vi "Get User Input.vi"(9 "Location":u32(ring) items=["None", "Austin, TX", "New York City, NY", "Chicago, IL"], 10 "Gender":enum32{"Radio Selection 1", "Radio Selection 2"}(radio), 11 "Name":string) -> (1 "Location":u32(ring) items=["Austin, TX", "New York City, NY", "Chicago, IL"], 2 "Gender":enum32{"Radio Selection 1", "Radio Selection 2"}(ring), 3 "Name":string)   [LabVIEW 2021, in "Dialog Box UI.lvlib"]
uses:
  Dialog Box UI.lvlib
panel:
  in  "Cancel":bool
  in  "OK":bool
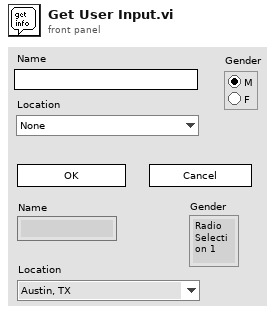
[diagram p1: front panel]
types:
  T1 = enum32{"None", "Radio Selection 1", "Radio Selection 2"}
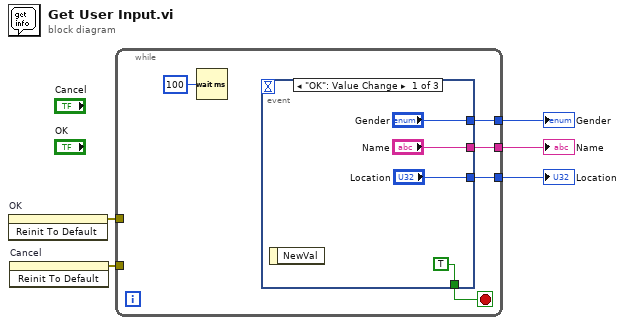
[diagram p0: block diagram]
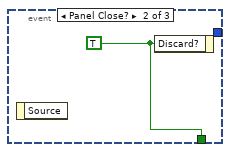
[diagram p2: hidden frame]
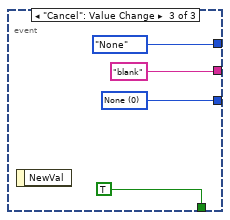
[diagram p3: hidden frame]
diagram:
  n1 = invoke on="OK" class="Bool" method="Reinit To Default"() -> (error out=w4:errorcluster)  [unwired: 3 in, 2 out]
  n2 = invoke on="Cancel" class="Bool" method="Reinit To Default"() -> (error out=w3:errorcluster)  [unwired: 3 in, 2 out]
  n3 = while {
    tunnel: [w10] -> w2
    tunnel: [w9] -> w5
    tunnel: [w8] -> w1
    tunnel: w4 -> [_]
    tunnel: w3 -> [_]
    stop <- w7 stop-if-true
    n4 = Wait (ms)(milliseconds to wait=u32 100) -> ()  [unwired: 1 out]
    n5 = event shown="[0] \"OK\": Value Change" {
      selector: _ -> [_ _ _]
      dyn-events: _ -> [_ _ _]
      timeout: _ -> [_ _ _]
      tunnel: [TRUE w15 TRUE] -> w7
      tunnel: ["Gender" _ T1."None" ("Gender")] -> w10
      tunnel: ["Name" _ "blank" ("Name")] -> w9
      tunnel: ["Location" _ w16] -> w8
      event "OK": Value Change {
        n6 = event-data() -> ()  [unwired: 2 out]
      }
      event Panel Close? {
        w15 = TRUE ("Discard?")
        n7 = event-data() -> ()  [unwired: 2 out]
        n8 = event-data("Discard?"=w15) -> ()  [unwired: 1 in, 1 out]
      }
      event "Cancel": Value Change {
        w16 = u32 0 items=["None", "Austin, TX", "New York City, NY", "Chicago, IL"] ("Location")
        n9 = event-data() -> ()  [unwired: 2 out]
      }
    }
  }
  "Name" <- w5
  "Gender" <- w2
  "Location" <- w1
